vi "EXA_issueCommand_EXAmple.vi"(8 "error in (no error)":errorcluster, 11 "command_EXAmple_Ctl":T1) -> (0 "error out":errorcluster, 2 "function return":i32, 3 "command_EXAmple_Ctl out":T1)   [LabVIEW 2016, in "SALLV_EXA.lvlib"]
doc: "int EXA_shm_issueCommand_EXAmpleLV(EXA_command_EXAmpleLV *command_EXAmple_Ctl );"
uses:
  SALLV_EXA.lvlib
  DataTypes/command_EXAmple.ctl
  SALLV_EXA.so
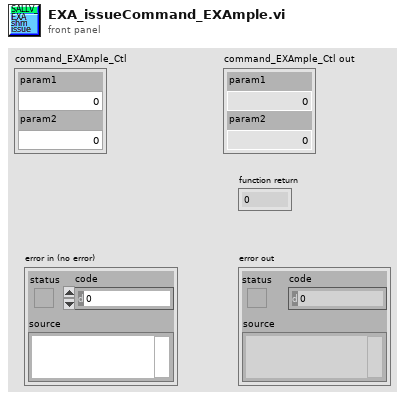
[diagram p1: front panel]
types:
  T1 = typedef "SALLV_EXA.lvlib/command_EXAmple.ctl" = cluster{"param1":dbl, "param2":dbl}
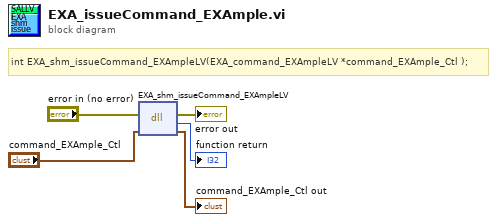
[diagram p0: block diagram]
diagram:
  # "int EXA_shm_issueCommand_EXAmpleLV(EXA_command_EXAmpleLV *command_EXAmple_Ctl );"
  n1 = dll-call lib="home/plotz/SALLV_EXA/SALLV_EXA.*" fn="EXA_shm_issueCommand_EXAmpleLV"(error in="error in (no error)", "command_EXAmple_Ctl"="command_EXAmple_Ctl") -> (error out=→"error out":errorcluster, →"function return":i32, "command_EXAmple_Ctl"=→"command_EXAmple_Ctl out":T1)  [unwired: 2 in, 1 out]
